vi "AssertVIFPStateCore.vi"(0 "VI Reference In":refnum<vi>, 1 "Label":string, 3 "Assert Only? (F)":bool, 5 "FP State":T1(ring), 11 "Error In":errorcluster, 12 "Assert Interval(10 ms)":u32=10, 13 "Timeout(5 sec)":dbl=5.0) -> (4 "VI Reference Out":refnum<vi>, 6 "Asserted Value":T1(ring), 15 "Error Out":errorcluster)   [LabVIEW 2016, in "Drona.lvlib" / "AssertVI.lvlib"]
doc: "Asserts the Front Panel State of the VI.\nThe input control name is given as a string , incase of path, use delimiters inbetween the path."
uses:
  AssertVI.lvlib
  <vilib>/addons/_JKI Toolkits/Caraya/classes/Assert/Assert True.vi
  <vilib>/addons/_JKI Toolkits/Caraya/classes/Assert/Assert.lvclass
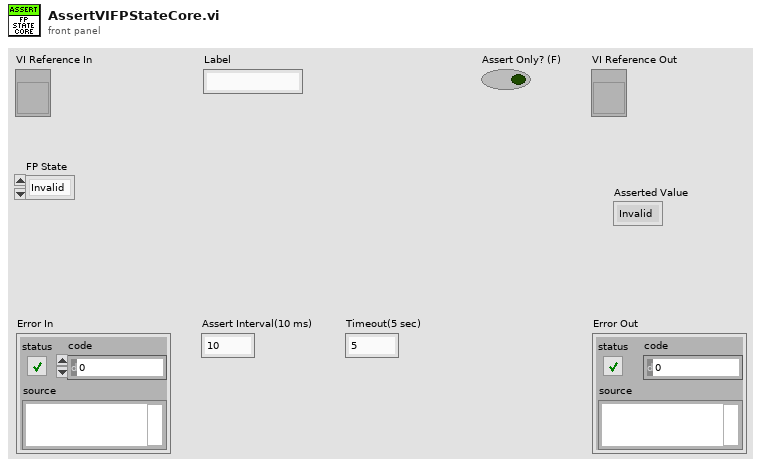
[diagram p1: front panel]
types:
  T1 = enum32{"Invalid", "Standard", "Closed", "Hidden", "Minimized", "Maximized"}
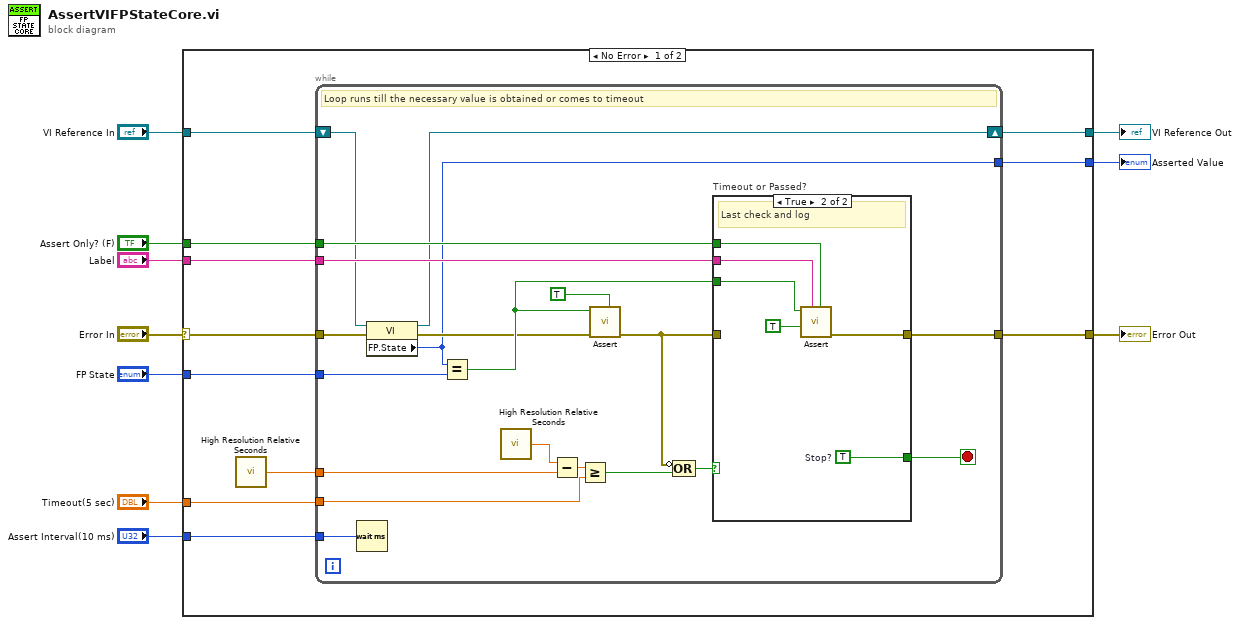
[diagram p0: block diagram]
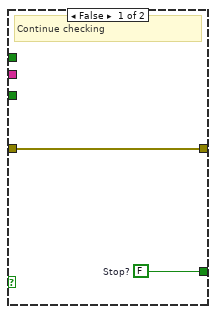
[diagram p2: hidden frame]
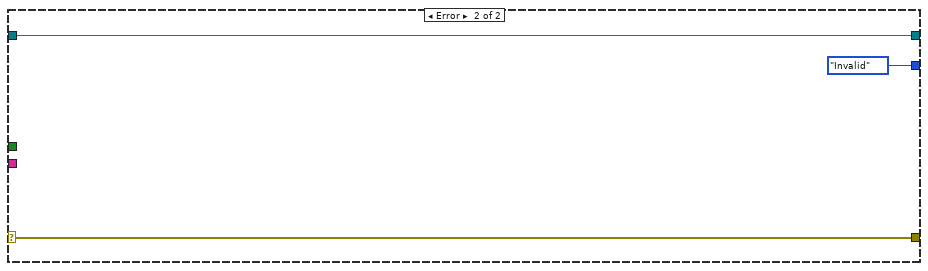
[diagram p3: hidden frame]
diagram:
  n1 = case shown="No Error" "Error In" {
    selector: "Error In" -> [w17 w52]
    tunnel: "Timeout(5 sec)" -> [w21 _]
    tunnel: [w20 w51] -> w9
    tunnel: [w13 w52] -> w8
    tunnel: "Assert Interval(10 ms)" -> [w19 _]
    tunnel: "Label" -> [w18 _]
    tunnel: "VI Reference In" -> [w16 w51]
    tunnel: "Assert Only? (F)" -> [w14 _]
    tunnel: "FP State" -> [w12 _]
    tunnel: [w11 T1."Invalid" ("Front Panel Window:State")] -> w1
    frame No Error {
      n2 = call <vilib>:"High Resolution Relative Seconds.vi"() -> ("relative seconds"=w15:dbl)
      n3 = while {
        tunnel: w21 -> [w40]
        tunnel: w15 -> [w41]
        tunnel: w17 -> [w36]
        tunnel: [w38] -> w13
        tunnel: w19 -> [w37]
        tunnel: w18 -> [w35]
        shift-right: [w24] -> w20
        shift-left: w16 -> [w25]
        tunnel: w14 -> [w34]
        tunnel: [w23] -> w11
        tunnel: w12 -> [w22]
        stop <- w39 stop-if-true
        # "Loop runs till the necessary value is obtained or comes to timeout"
        n4 = Wait (ms)(milliseconds to wait=w37) -> ()  [unwired: 1 out]
        n5 = property class="VI"(reference=w25, error in=w36) -> (reference out=w24:refnum<vi>, error out=w26:errorcluster, "FP.State"=w23:T1)
        n6 = Equal?(x=w23, y=w22) -> (x = y?=w27:bool)
        n7 = call <vilib>:"High Resolution Relative Seconds.vi"() -> ("relative seconds"=w33:dbl)
        n8 = Subtract(x=w33, y=w41) -> (x-y=w32:dbl)
        n9 = Greater Or Equal?(x=w32, y=w40) -> (x >= y?=w31:bool)
        n10 = call-poly <vilib>:"Assert.vi"("Assert Only? (F)"=TRUE, "error in (no error)"=w26, "True?"=w27) -> ("error out"=w30:errorcluster)  [unwired: 7 in, 1 out]
        n11 = Compound Arithmetic op=OR(invert w30, w31) -> (w29:bool)
        n12 = case "Timeout or Passed?" shown="True" w29 {
          tunnel: w30 -> [w43 _]
          tunnel: w27 -> [_ w48]
          tunnel: w35 -> [_ w49]
          tunnel: [w43 w47] -> w38
          tunnel: [w42 w46] -> w39
          tunnel: w34 -> [_ w44]
          frame False {
            w42 = FALSE  # Stop?
            # "Continue checking"
          }
          frame True {
            w46 = TRUE  # Stop?
            # "Last check and log"
            n13 = call-poly <vilib>:"Assert.vi"("Assert Only? (F)"=w44, "Label"=w49, "Register with caller test (F)"=TRUE, "True?"=w48) -> ("error out"=w47:errorcluster)  [unwired: 6 in, 1 out]
          }
        }
      }
    }
    frame Error {
    }
  }
  "Error Out" <- w8
  "VI Reference Out" <- w9
  "Asserted Value" <- w1
